vi "WriteJointPositionRegister.vi"(8 "Value":dbl[](array[numeric]), 9 "index":i32, 10 "Snpx":refnum<k24>, 11 "error in":errorcluster) -> (3 "error out":errorcluster)   [LabVIEW 2023, in "UnderAutomation.Fanuc.lvlib"]
uses:
  UnderAutomation.Fanuc.lvlib
  C:/Users/fg/Documents/Fanuc.vi/LabVIEW_2024/UnderAutomation.Fanuc/lib/UnderAutomation.Fanuc.dll
  LabVIEW_2024/UnderAutomation.Fanuc/lib/UnderAutomation.Fanuc.dll
panel:
  in  "jointsPosition":refnum<k24>
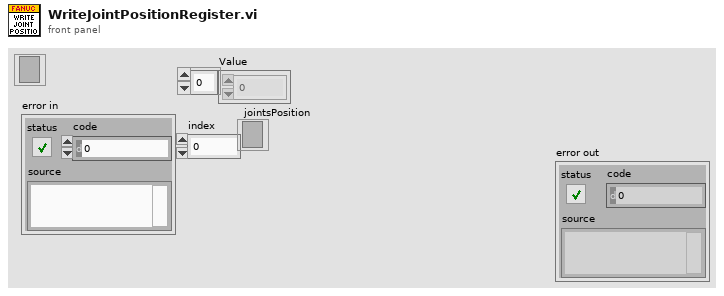
[diagram p1: front panel]
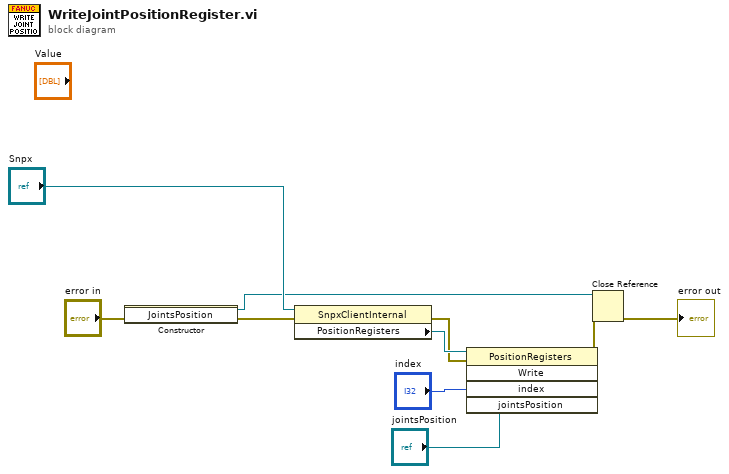
[diagram p0: block diagram]
diagram:
  n1 = constructor class="JointsPosition"(error in="error in") -> (reference out=w3:refnum<k24>, error out=w5:errorcluster)  [unwired: 2 in, 1 out]
  n2 = property class="SnpxClientInternal"(reference="Snpx", error in=w5) -> (error out=w8:errorcluster, "PositionRegisters"=w9:refnum<k24>)  [unwired: 1 out]
  n3 = invoke class="PositionRegisters" method="Write"(reference=w9, error in=w8, "index"="index", "jointsPosition"="jointsPosition") -> (error out=w4:errorcluster)  [unwired: 1 in, 4 out]
  n4 = Close Reference(reference=w3, error in (no error)=w4) -> (error out=→"error out":errorcluster)
